vi "Parse Headers.vi"(11 "HTTP Headers":string) -> (3 "Response Headers":cluster{"header":string, "value":string}[](array[cluster]))   [LabVIEW 2018, in "REST Client_JKI.lvlib" / "Response Headers.lvclass"]
uses:
  Response Headers.lvclass
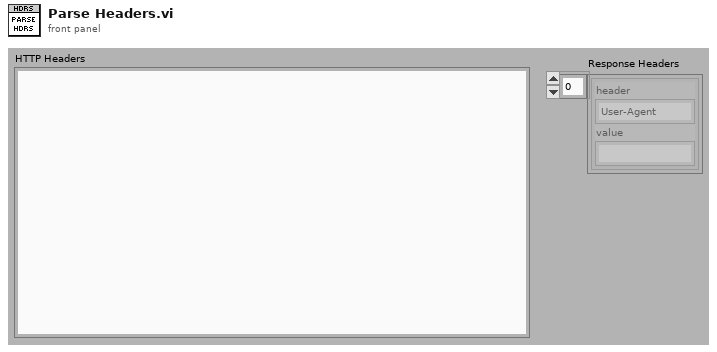
[diagram p1: front panel]
types:
  T1 = cluster{"trimmed string":string, "trimmed string":string}
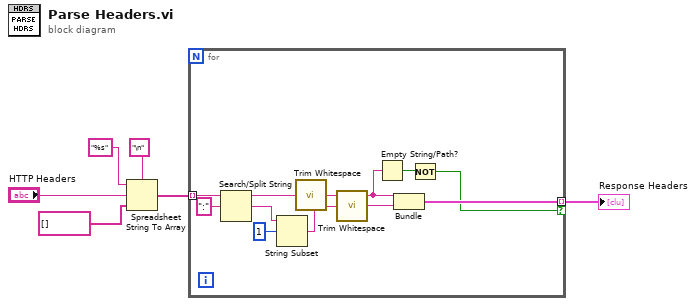
[diagram p0: block diagram]
diagram:
  n1 = Spreadsheet String To Array(delimiter (Tab)="\n", format string="%s", spreadsheet string="HTTP Headers", array type (2D Dbl)=string[] []) -> (array=w2:string[])
  n2 = for {
    tunnel: w2 -> [w17] mode=indexing
    tunnel: [w14] -> w1 mode=indexing if=w9
    n3 = Search/Split String(string=w17, search string/char (-)=":") -> (substring before match=w8:string, match + rest of string=w13:string)  [unwired: 1 in, 1 out]
    n4 = String Subset(string=w13, offset (0)=1) -> (substring=w11:string)  [unwired: 1 in]
    n5 = call <vilib>:"Trim Whitespace.vi"("string"=w8) -> ("trimmed string"=w7:string)  [unwired: 1 in]
    n6 = call <vilib>:"Trim Whitespace.vi"("string"=w11) -> ("trimmed string"=w15:string)  [unwired: 1 in]
    n7 = Empty String/Path?(string/path=w7) -> (empty?=w10:bool)
    n8 = Bundle("trimmed string"=w7, "trimmed string"=w15) -> (w14:T1)  [unwired: 1 in]
    n9 = Not(x=w10) -> (.not. x?=w9:bool)
  }
  "Response Headers" <- w1
